vi "GetProperties.vi"(8 "error in":errorcluster, 11 "GraphChart in":refnum<class "GraphChart.lvclass">) -> (0 "error out":errorcluster, 3 "GraphChart out":refnum<class "GraphChart.lvclass">)   [LabVIEW 2014, in "Raspberry Pi Compatible Compiler for LabVIEW.lvlib" / "GraphChart.lvclass"]
uses:
  GraphChart.lvclass
  GraphChart.lvclass/GraphChart.ctl
  Control/Control.lvclass
  GraphScale/GraphScale.lvclass
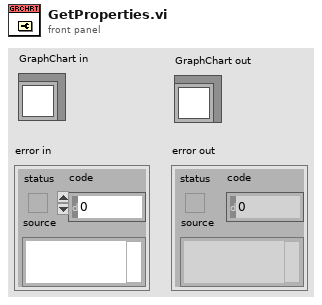
[diagram p1: front panel]
types:
  T1 = typedef "LVRectTypeDef.ctl" = cluster{"Left":i16, "Top":i16, "Right":i16, "Bottom":i16}
  T2 = typedef "LVForegroundBackgroundColorsTypeDef.ctl" = cluster{"FG Color":u32, "BG Color":u32}
  T3 = typedef "LVBoundsTypeDef.ctl" = cluster{"Width":u32, "Height":u32}
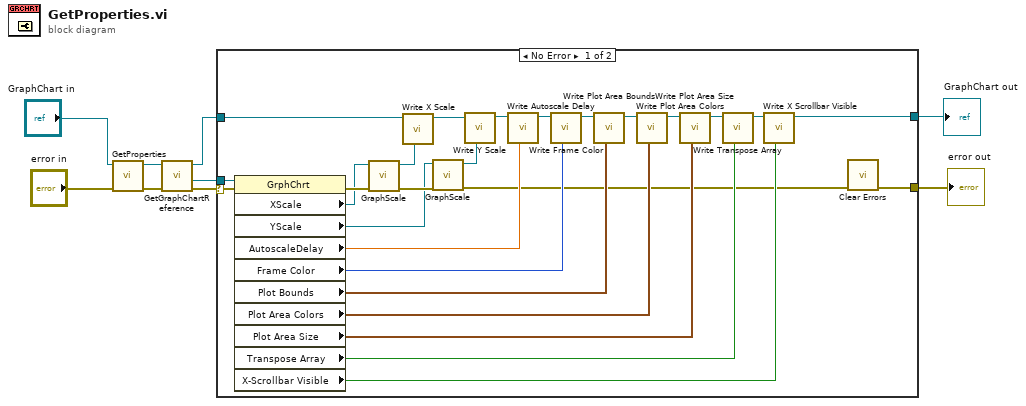
[diagram p0: block diagram]
diagram:
  n1 = call-parent "GetProperties.vi"("error in"="error in", "Control in"="GraphChart in") -> ("error out"=w7:errorcluster, "Control out"=w6:refnum<class "GraphChart.lvclass">)  [unwired: 8 in]
  n2 = call "GetGraphChartReference.vi"("error in"=w7, "GraphChart in"=w6) -> ("error out"=w5:errorcluster, "graph scale reference"=w4:refnum<vi>, "GraphChart out"=w3:refnum<class "GraphChart.lvclass">)  [unwired: 7 in]
  n3 = case shown="No Error" w5 {
    selector: w5 -> [w35 w37]
    tunnel: w4 -> [w36 _]
    tunnel: w3 -> [w14 w38]
    tunnel: [w22 w38] -> w2
    tunnel: [w10 w37] -> w1
    frame No Error {
      n4 = property class="GrphChrt"(reference=w36, error in=w35) -> (error out=w19:errorcluster, "XScale"=w18:refnum<vi>, "YScale"=w16:refnum<vi>, "AutoscaleDelay"=w34:sgl, "Frame Color"=w33:u32, "Plot Bounds"=w32:T1, "Plot Area Colors"=w26:T2, "Plot Area Size"=w25:T3, "Transpose Array"=w24:bool, "X-Scrollbar Visible"=w21:bool)  [unwired: 1 out]
      n5 = call "GraphScale.vi"("error in"=w19, "Gen Refnum"=w18) -> ("error out"=w17:errorcluster, "GraphScale out"=w15:refnum<class "GraphScale.lvclass">)  [unwired: 8 in]
      n6 = call "Write X Scale.vi"("X scale"=w15, "GraphChart in"=w14) -> ("GraphChart out"=w13:refnum<class "GraphChart.lvclass">)  [unwired: 7 in]
      n7 = call "GraphScale.vi"("error in"=w17, "Gen Refnum"=w16) -> ("error out"=w11:errorcluster, "GraphScale out"=w12:refnum<class "GraphScale.lvclass">)  [unwired: 8 in]
      n8 = call "Write Y Scale.vi"("Y scale"=w12, "GraphChart in"=w13) -> ("GraphChart out"=w20:refnum<class "GraphChart.lvclass">)  [unwired: 7 in]
      n9 = call "Write Autoscale Delay.vi"("Autoscale Delay"=w34, "GraphChart in"=w20) -> ("GraphChart out"=w29:refnum<class "GraphChart.lvclass">)  [unwired: 7 in]
      n10 = call "Write Frame Color.vi"("Frame Color"=w33, "GraphChart in"=w29) -> ("GraphChart out"=w31:refnum<class "GraphChart.lvclass">)  [unwired: 7 in]
      n11 = call "Write Plot Area Bounds.vi"("Plot Area Bounds"=w32, "GraphChart in"=w31) -> ("GraphChart out"=w30:refnum<class "GraphChart.lvclass">)  [unwired: 7 in]
      n12 = call "Write Plot Area Colors.vi"("Plot Area Colors"=w26, "GraphChart in"=w30) -> ("GraphChart out"=w28:refnum<class "GraphChart.lvclass">)  [unwired: 7 in]
      n13 = call "Write Plot Area Size.vi"("Plot Area Size"=w25, "GraphChart in"=w28) -> ("GraphChart out"=w27:refnum<class "GraphChart.lvclass">)  [unwired: 7 in]
      n14 = call "Write Transpose Array.vi"("Transpose Array"=w24, "GraphChart in"=w27) -> ("GraphChart out"=w23:refnum<class "GraphChart.lvclass">)  [unwired: 7 in]
      n15 = call "Write X Scrollbar Visible.vi"("X Scrollbar Visible"=w21, "GraphChart in"=w23) -> ("GraphChart out"=w22:refnum<class "GraphChart.lvclass">)  [unwired: 7 in]
      n16 = call <vilib>:"Clear Errors.vi"("error in (no error)"=w11) -> ("error out"=w10:errorcluster)  [unwired: 5 in, 1 out]
    }
    frame Error {
    }
  }
  "error out" <- w1
  "GraphChart out" <- w2
